vi "setId.vi"(8 "error in (no error)":errorcluster, 10 "ID":i32, 11 "pCircle in":refnum<class "pCircle.lvclass">) -> (0 "error out":errorcluster, 3 "pCircle out":refnum<class "pCircle.lvclass">)   [LabVIEW 2017, in "pCircle.lvclass"]
uses:
  pCircle.lvclass
  pCircle.lvclass/pCircle.ctl
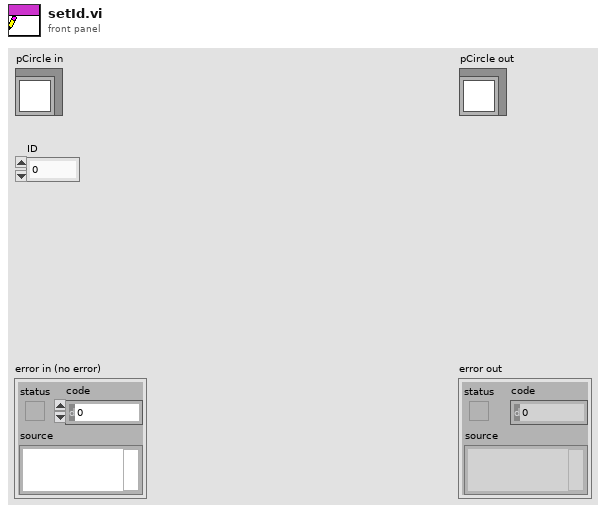
[diagram p1: front panel]
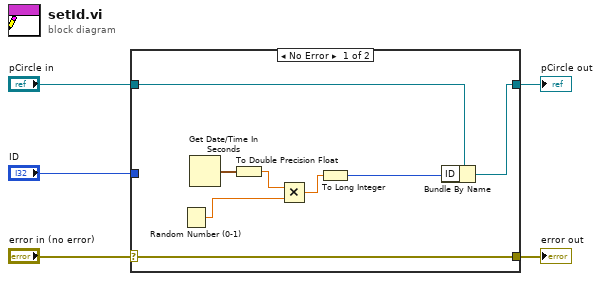
[diagram p0: block diagram]
diagram:
  n1 = case shown="No Error" "error in (no error)" {
    selector: "error in (no error)" -> [w13 w14]
    tunnel: [w13 w14] -> w4
    tunnel: [w11 w15] -> w2
    tunnel: "pCircle in" -> [w12 w15]
    tunnel: "ID" -> [_ _]
    frame No Error {
      n2 = Random Number (0-1)() -> (number: 0 to 1=w8:dbl)
      n3 = Get Date/Time In Seconds() -> (seconds since 1Jan1904=w10:timestamp)
      n4 = To Double Precision Float(number=w10) -> (double precision float=w9:dbl)
      n5 = Multiply(x=w9, y=w8) -> (x*y=w7:dbl)
      n6 = To Long Integer(number=w7) -> (32bit integer=w6:i32)
      n7 = Bundle By Name(cluster=w12, "ID"=w6) -> (w11:refnum<class "pCircle.lvclass">)
    }
    frame Error {
    }
  }
  "error out" <- w4
  "pCircle out" <- w2
